vi "Parse Channels.vi"(7 "Rx? (T:True, F: False (Tx))":bool, 8 "error in (no error)":errorcluster, 9 "Specified Channel Ref List":T1[](array[typedef]) format="%.0x", 10 "Section GUID":string, 11 "Device Reference in":T1 format="%.0x") -> (0 "error out":errorcluster, 2 "Channel Data []":T2[](array[typedef]) {"Labels Settings"."Label Timestamp Channel Data Reference" format="%.0x"; "Labels Settings"."Label Disable/Trigger Channel Reference" format="%.0x"; "Labels Settings"."Word"."Param Setting"."Item Refs" format="%.0x"; "Labels Settings"."Word"."Param Setting"."Num Bits" min=1 max=32; "Labels Settings"."Word"."Param Setting"."Start Bit" min=8 max=31; "Labels Settings"."Label" format="%.0o"}, 3 "Device Reference out":T1 format="%.0x")   [LabVIEW 2016, in "Ballard Arinc-429 System Explorer.lvlib"]
uses:
  Ballard Arinc-429 System Explorer.lvlib
  <vilib>/NI VeriStand/Custom Device Tools/Custom Device Utility Library/Custom Device Utility Library.lvlib
  <vilib>/NI VeriStand/Custom Device API/Custom Device API.lvlib
  Shared/Controls and Global/Number of Bits.ctl
  Shared/Ballard Arinc-429 Shared.lvlib
  Shared/Controls and Global/Start Bit.ctl
  Shared/Controls and Global/transferPeriod.ctl
  Shared/Controls and Global/Label.ctl
  Shared/Controls and Global/RT Label Settings.ctl
  Shared/Controls and Global/RT HW Channel.ctl
  Shared/Controls and Global/Global.vi
  <vilib>/NI Veristand/Custom Device Tools/Custom Device Utility Library/NI VeriStand - Search for Item by GUID.vi
  <vilib>/NI Veristand/Custom Device API/Get Item Property (U16).vi
  Shared/Controls and Global/RT Param Setting.ctl
  Shared/Controls and Global/RT Word Settings.ctl
  Shared/Controls and Global/TransferType.ctl
  <vilib>/NI Veristand/Custom Device API/Data Reference.ctl
  <vilib>/NI Veristand/Custom Device API/Block Data Reference.ctl
  <vilib>/NI Veristand/Custom Device API/Custom Device Item Ref.ctl
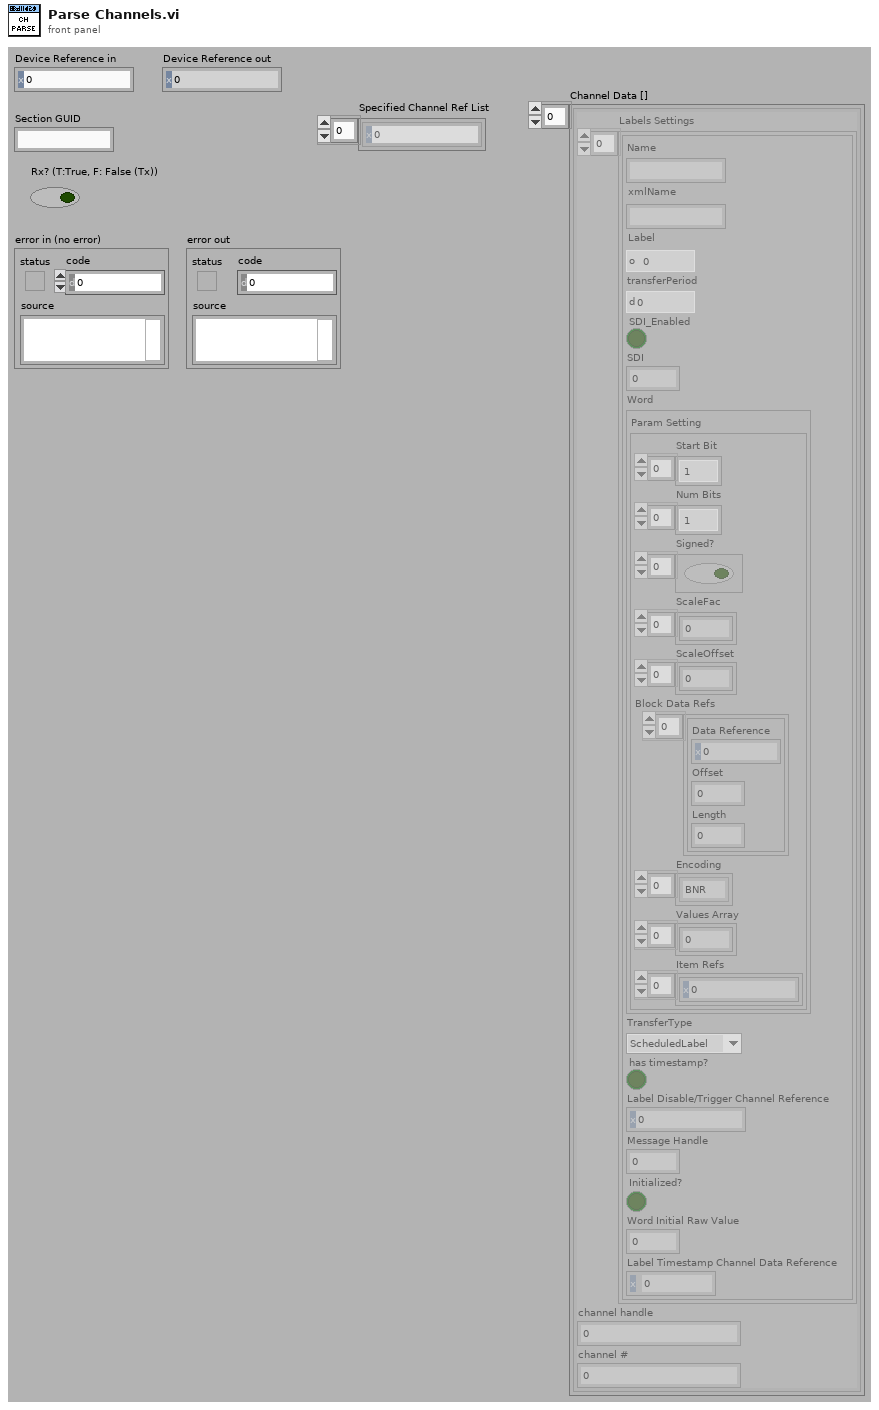
[diagram p1: front panel]
types:
  T1 = typedef "Custom Device API.lvlib/Custom Device Item Ref.ctl" = u64
  T2 = typedef "Ballard Arinc-429 Shared.lvlib/RT HW Channel.ctl" = cluster{"Labels Settings":T3[], "channel handle":u64, "channel #":u16}
  T3 = typedef "Ballard Arinc-429 Shared.lvlib/RT Label Settings.ctl" = cluster{"Name":string, "xmlName":string, "Label":T4, "transferPeriod":T5, "SDI_Enabled":bool, "SDI":u8, "Word":T6, "TransferType":T12, "has timestamp?":bool, "Label Disable/Trigger Channel Reference":T1, "Message Handle":u64, "Initialized?":bool, "Word Initial Raw Value":u32, "Label Timestamp Channel Data Reference":T11}
  T4 = typedef "Ballard Arinc-429 Shared.lvlib/Label.ctl" = u8
  T5 = typedef "Ballard Arinc-429 Shared.lvlib/transferPeriod.ctl" = u32
  T6 = typedef "Ballard Arinc-429 Shared.lvlib/RT Word Settings.ctl" = cluster{"Param Setting":T7}
  T7 = typedef "Ballard Arinc-429 Shared.lvlib/RT Param Setting.ctl" = cluster{"Start Bit":T8[], "Num Bits":T9[], "Signed?":bool[], "ScaleFac":dbl[], "ScaleOffset":dbl[], "Block Data Refs":T10[], "Encoding":enum16{"BNR", "BCD", "Discrete"}[], "Values Array":dbl[], "Item Refs":T1[]}
  T8 = typedef "Ballard Arinc-429 Shared.lvlib/Start Bit.ctl" = i32
  T9 = typedef "Ballard Arinc-429 Shared.lvlib/Number of Bits.ctl" = i32
  T10 = typedef "Custom Device API.lvlib/Block Data Reference.ctl" = cluster{"Data Reference":T11, "Offset":u64, "Length":u64}
  T11 = typedef "Custom Device API.lvlib/Data Reference.ctl" = i32
  T12 = typedef "Ballard Arinc-429 Shared.lvlib/TransferType.ctl" = enum16{"ScheduledLabel", "Acyclic", "Block", "Strobe"}
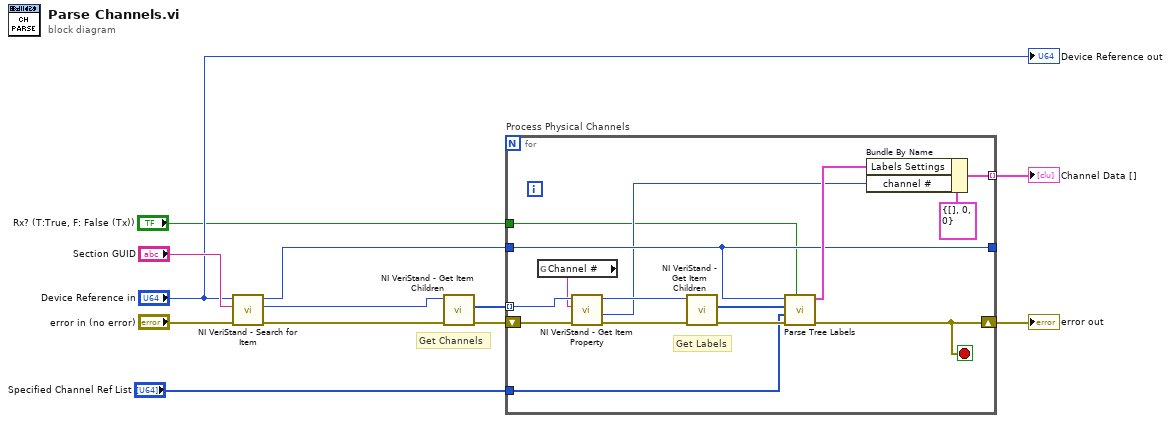
[diagram p0: block diagram]
diagram:
  # "Get Channels"
  n1 = call-poly <vilib>:"NI VeriStand - Search for Item.vi"("error in"="error in (no error)", "Item GUID"="Section GUID", "Section Ref in"="Device Reference in") -> ("error out"=w7:errorcluster, "Item Ref"=w8:T1, "Section Ref out"=w12:T1)  [unwired: 5 in, 1 out]
  n2 = call <vilib>:"NI VeriStand - Get Item Children.vi"("error in (no error)"=w7, "Item Ref in"=w8) -> ("error out"=w11:errorcluster, "Child Refs"=w10:T1[])  [unwired: 6 in, 2 out]
  n3 = for "Process Physical Channels" {
    tunnel: w10 -> [w21] mode=indexing
    tunnel: w12 -> [w19]
    tunnel: [w25] -> w5 mode=indexing
    shift-right: [w15] -> w1
    shift-left: w11 -> [w23]
    tunnel: [w19] -> _
    tunnel: "Specified Channel Ref List" -> [w14]
    tunnel: "Rx? (T:True, F: False (Tx))" -> [w13]
    stop <- w15 stop-if-true
    # "Get Labels"
    n4 = global read "Global.vi" "Channel #"() -> (w17:string)
    n5 = call-poly <vilib>:"NI VeriStand - Get Item Property.vi"("error in (no error)"=w23, "Property Name"=w17, "Item Ref in"=w21) -> ("error out"=w22:errorcluster, "Value"=w16:u16, "Item Ref out"=w20:T1)  [unwired: 5 in, 1 out]
    n6 = call <vilib>:"NI VeriStand - Get Item Children.vi"("error in (no error)"=w22, "Item Ref in"=w20) -> ("error out"=w24:errorcluster, "Child Refs"=w18:T1[])  [unwired: 6 in, 2 out]
    n7 = call "Parse Tree Labels.vi"("Rx? (T:True, F: False (Tx))"=w13, "error out"=w24, "Specified Channel Ref List"=w14, "Label Refs"=w18, "Custom Device Ref"=w19) -> ("error out"=w15:errorcluster, "Label data"=w26:T3[])  [unwired: 5 in]
    n8 = Bundle By Name(cluster=T2 {"Labels Settings"=[], "channel handle"=0, "channel #"=0} ("HW Channel"), "Labels Settings"=w26, "channel #"=w16) -> (w25:T2)
  }
  "Channel Data []" <- w5
  "error out" <- w1
  "Device Reference out" <- "Device Reference in"
